vi "Update plot from list.vi"(8 "error in (no error)":errorcluster, 11 "Cap Bank Server in":refnum<class "Cap Bank Server.lvclass">) -> (0 "error out":errorcluster, 3 "Cap Bank Server out":refnum<class "Cap Bank Server.lvclass">)   [LabVIEW 2015, in "Cap Bank Server.lvclass"]
uses:
  Cap Bank Server.lvclass
  Cap Bank Server.lvclass/Cap Bank Server.ctl
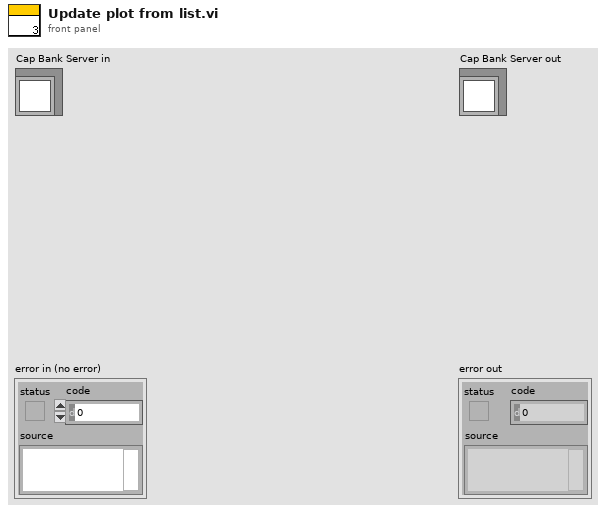
[diagram p1: front panel]
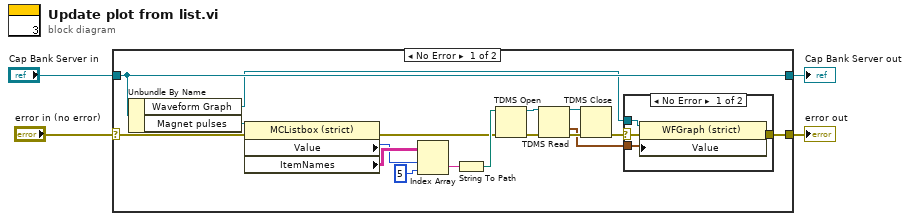
[diagram p0: block diagram]
diagram:
  n1 = case shown="No Error" "error in (no error)" {
    selector: "error in (no error)" -> [w15 w28]
    tunnel: [w6 w28] -> w3
    tunnel: [w21 w27] -> w1
    tunnel: "Cap Bank Server in" -> [w21 w27]
    frame No Error {
      n2 = Unbundle By Name(w21) -> ("Waveform Graph"=w8:refnum<vi>, "Magnet pulses"=w20:refnum<vi>)
      n3 = property class="MCListbox (strict)"(reference=w20, error in=w15) -> (error out=w11:errorcluster, "Value"=w18:i32, "ItemNames"=w19:string[][])  [unwired: 1 out]
      n4 = Index Array(array=w19, index (row)=w18, index (col)=5 ("disabled index (col)")) -> (element=w16:string)
      n5 = String To Path(string=w16) -> (path=w14:path)
      n6 = TDMS Open(8:w11, 11:w14) -> (0:w12:errorcluster, 3:w13:refnum<k34>)  [unwired: 5 in]
      n7 = TDMS Read(0:w13, 11:w12) -> (4:w5:refnum<k34>, 10:w7:waveform(dbl)[], 15:w10:errorcluster)  [unwired: 6 in, 3 out]
      n8 = TDMS Close(8:w10, 11:w5) -> (0:w9:errorcluster)  [unwired: 1 out]
      n9 = case shown="No Error" w9 {
        selector: w9 -> [w24 w26]
        tunnel: w8 -> [w25 _]
        tunnel: w7 -> [w23 _]
        tunnel: [w22 w26] -> w6
        frame No Error {
          n10 = property class="WFGraph (strict)"(reference=w25, error in=w24, "Value"=w23) -> (error out=w22:errorcluster)  [unwired: 1 out]
        }
        frame Error {
        }
      }
    }
    frame Error {
    }
  }
  "error out" <- w3
  "Cap Bank Server out" <- w1
